vi "TestConnection_3.vi"() -> ()   [LabVIEW 2024]
uses:
  <vilib>/LabVIEW Open Source Project/MQTT Control Packets/Control Packets/CONNECT/ConnectFlags -- cluster.ctl
  <vilib>/LabVIEW Open Source Project/MQTT Control Packets/Control Packets/CONNACK/Connect Return Code -- enum.ctl
  <vilib>/LabVIEW Open Source Project/MQTT Control Packets/Control Packets/SUBSCRIBE/Topic Subscription -- cluster.ctl
  <vilib>/LabVIEW Open Source Project/MQTT Control Packets/Control Packets/ControlPacket/QualityOfService -- enum.ctl
  <vilib>/LabVIEW Open Source Project/MQTT Control Packets/Control Packets/SUBACK/Subscription Success Code.ctl
  <vilib>/LabVIEW Open Source Project/MQTT Secured TCP Connection/Connection.SecuredTCP/Connection.TCP-TLS.lvclass
  C:/Program Files (x86)/National Instruments/LabVIEW 2024/vi.lib/LabVIEW Open Source Project/Connection/Connection/Connection.lvclass
  <vilib>/LabVIEW Open Source Project/MQTT Client/Client class/Client.lvclass
  C:/Program Files (x86)/National Instruments/LabVIEW 2024/vi.lib/LabVIEW Open Source Project/MQTT Connection/MQTT_Base/Base Class/MQTT_Base.lvclass
  <vilib>/LabVIEW Open Source Project/MQTT Connection/MQTT_Base/Base Class/MQTT_Base.lvclass
  <vilib>/LabVIEW Open Source Project/MQTT Control Packets/Control Packets/CONNECT/CONNECT.lvclass
  <vilib>/LabVIEW Open Source Project/MQTT Control Packets/Control Packets/CONNACK/CONNACK.lvclass
  <vilib>/LabVIEW Open Source Project/MQTT Control Packets/Control Packets/ControlPacket/ControlPacket.lvclass
  <vilib>/LabVIEW Open Source Project/MQTT Control Packets/Control Packets/SUBSCRIBE/SUBSCRIBE.lvclass
  <vilib>/LabVIEW Open Source Project/MQTT Control Packets/Control Packets/SUBACK/SUBACK.lvclass
panel:
  out "SUBACK Packet ID":u16 format="%04x"
  out "Subscription Success":T1[](array[typedef])
  in  "Topic Subscriptions":T3[](array[typedef])
  in  "Message":string="PID=30,0.1,0"
  out "Published":bool=TRUE
  in  "Topic Name (empty: Payload name)":string="commands/topic"
  out "Auth Client?":bool
  in  "password":string
  in  "Client Private Key":path=path "C:/Users/viasl/Desktop/Skole/IIA3220/IIA3220/TestCerts/mqtt-client-key.pem"
  in  "Client X.509 Certificate":path=path "C:/Users/viasl/Desktop/Skole/IIA3220/IIA3220/TestCerts/mqtt-client-cert.crt"
  out "Ready for SSL":bool=TRUE
  in  "Server X.509 Certificate":path=path "C:/Users/viasl/Desktop/Skole/IIA3220/IIA3220/TestCerts/isrgrootx1.pem"
  in  "Hostname":string="ce06b4f8ae4542a08357c542c4882795.s1.eu.hivemq.cloud"
  out "timed out":bool
  in  "remote port (80)":u16=8883
  out "error out":errorcluster
  out "Return Code":T4
  in  "Connect Flags":T5={"Reserved"=FALSE, "Clean Session"=TRUE, "Will Flag"=FALSE, "Will QoS 1"=FALSE, "Will QoS 2"=FALSE, "Will Retain"=FALSE, "Password Flag"=TRUE, "User Name Flag"=TRUE}
  in  "Payload":T6={"Will Topic"="", "Will Message"="", "Username"="CustomerClient", "Password"="CustomerClient1"}
  # "Root CA Certificate"
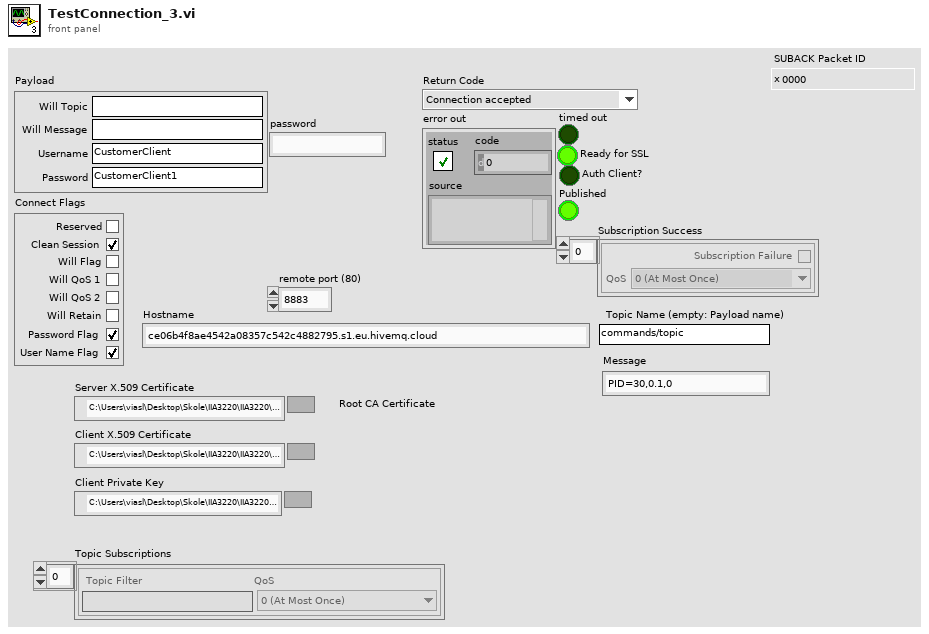
[diagram p1: front panel]
types:
  T1 = typedef "MQTT_Control_Packets.lvlib/SUBACK.lvclass/Subscription Success Code.ctl" = cluster{"Subscription Failure":bool, "QoS":T2}
  T2 = typedef "MQTT_Control_Packets.lvlib/ControlPacket.lvclass/QualityOfService -- enum.ctl" = enum16{"0 (At Most Once)", "1 (At Least Once)", "2 (Exactly Once)"}
  T3 = typedef "MQTT_Control_Packets.lvlib/SUBSCRIBE.lvclass/Topic Subscription -- cluster.ctl" = cluster{"Topic Filter":string, "QoS":T2}
  T4 = typedef "MQTT_Control_Packets.lvlib/CONNACK.lvclass/Connect Return Code -- enum.ctl" = enum16{"Connection accepted", "Unacceptable protocol version", "Identifier Rejected", "Server Unavailable", "Bad Username or Password", "Not Authorized"}
  T5 = typedef "MQTT_Control_Packets.lvlib/CONNECT.lvclass/ConnectFlags -- cluster.ctl" = cluster{"Reserved":bool, "Clean Session":bool, "Will Flag":bool, "Will QoS 1":bool, "Will QoS 2":bool, "Will Retain":bool, "Password Flag":bool, "User Name Flag":bool}
  T6 = cluster{"Will Topic":string, "Will Message":string, "Username":string, "Password":string}
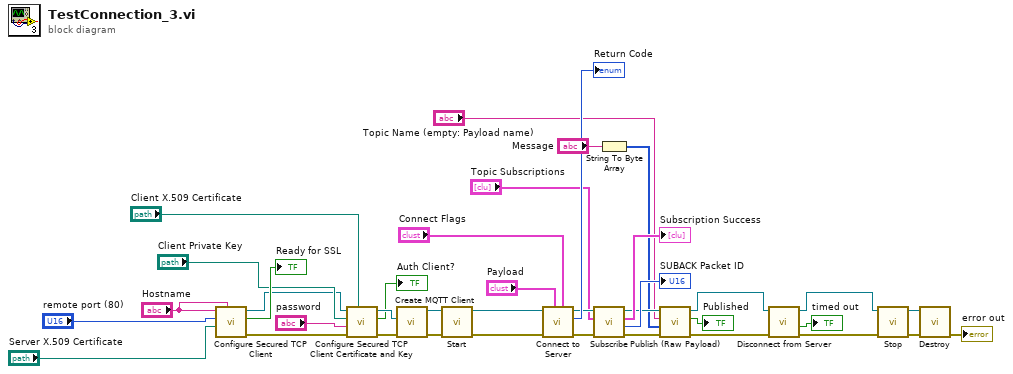
[diagram p0: block diagram]
diagram:
  n1 = call <vilib>:"Configure Secured TCP Client.vi"("Hostname"="Hostname", "Server X.509 Certificate"="Server X.509 Certificate", "remote port (443)"="remote port (80)", "address (localhost)"="Hostname") -> ("error out"=w16:errorcluster, "Ready for SSL"=→"Ready for SSL":bool, "Secured TCP Connection"=w15:refnum<class "Connection.TCP-TLS.lvclass">)  [unwired: 5 in]
  n2 = call <vilib>:"Configure Secured TCP Client Certificate and Key.vi"("Client X.509 Certificate"="Client X.509 Certificate", "error in (no error)"=w16, "password"="password", "Client Private Key"="Client Private Key", "Connection.TCP-TLS in"=w15) -> ("error out"=w22:errorcluster, "Auth Client?"=→"Auth Client?":bool, "Connection.TCP-TLS out"=w23:refnum<class "Connection.TCP-TLS.lvclass">)  [unwired: 4 in]
  n3 = call <vilib>:"Create MQTT Client.vi"("error in (no error)"=w22, "Connection Configuration"=w23) -> ("error out"=w36:errorcluster, "Client out"=w35:refnum<class "Client.lvclass">)  [unwired: 8 in]
  n4 = call <vilib>:"Start.vi"("error in (no error)"=w36, "MQTT_Base in"=w35) -> ("error out"=w33:errorcluster, "MQTT_Base out"=w34:refnum<class "Client.lvclass">)  [unwired: 7 in, 1 out]
  n5 = call <vilib>:"Connect to Server.vi"("Connect Flags"="Connect Flags", "Payload"="Payload", "error in (no error)"=w33, "Client in"=w34) -> ("error out"=w13:errorcluster, "Return Code"=→"Return Code":T4, "Client out"=w12:refnum<class "Client.lvclass">)  [unwired: 4 in, 1 out]
  n6 = call <vilib>:"Subscribe.vi"("error in (no error)"=w13, "Topic Subscriptions"="Topic Subscriptions", "MQTT_Base in"=w12) -> ("error out"=w5:errorcluster, "SUBACK Packet ID"=→"SUBACK Packet ID":u16, "Subscription Success"=→"Subscription Success":T1[], "MQTT_Base out"=w4:refnum<class "Client.lvclass">)  [unwired: 5 in]
  n7 = String To Byte Array(string="Message") -> (unsigned byte array=w1:u8[])
  n8 = call <vilib>:"Publish (Raw Payload).vi"("error in (no error)"=w5, "Binary Payload"=w1, "Topic Name"="Topic Name (empty: Payload name)", "Client in"=w4) -> ("error out"=w6:errorcluster, "Published"=→"Published":bool, "Client out"=w7:refnum<class "Client.lvclass">)  [unwired: 5 in]
  n9 = call <vilib>:"Disconnect from Server.vi"("error in (no error)"=w6, "Client in"=w7) -> ("error out"=w30:errorcluster, "timed out"=→"timed out":bool, "Client out"=w31:refnum<class "Client.lvclass">)  [unwired: 7 in]
  n10 = call <vilib>:"Stop.vi"("error in (no error)"=w30, "MQTT_Base in"=w31) -> ("error out"=w29:errorcluster, "MQTT_Base out"=w28:refnum<class "Client.lvclass">)  [unwired: 7 in, 1 out]
  n11 = call <vilib>:"Destroy.vi"("error in (no error)"=w29, "MQTT_Base in"=w28) -> ("error out"=→"error out":errorcluster)  [unwired: 8 in, 1 out]
